vi "Acquisition.vi"(5 "Mode":enum16{"Grab", "Snap"}(ring), 6 "Image Type":T1 items=["Grayscale (U8)", "Grayscale (I16)", "Grayscale (SGL)", "Complex (CSG)", "RGB (U32)", "HSL (U32)", "RGB (U64)", "Grayscale (U16)"], 8 "Error In":errorcluster, 11 "Session In":T3) -> (0 "Error Out":errorcluster, 2 "Image Out":T2, 3 "IMAQdx Session Out":T3)   [LabVIEW 2020]
uses:
  <vilib>/userdefined/High Color/IMAQdx.ctl
  <vilib>/vision/Image Controls.llb/IMAQ Image.ctl
  <vilib>/vision/driver/IMAQdx.llb/IMAQdx Camera Control Mode.ctl
  <vilib>/vision/driver/NI_Vision_Acquisition_Software.lvlib
  <resource>/objmgr/imaqdx.rc
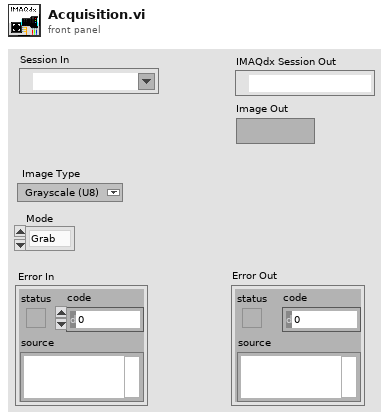
[diagram p1: front panel]
types:
  T1 = typedef "Image Type" = u32
  T2 = typedef "IMAQ Image.ctl" = refnum<image>
  T3 = typedef "IMAQdx.ctl" = refnum<k21>
  T4 = typedef "NI_Vision_Acquisition_Software.lvlib/IMAQdx Camera Control Mode.ctl" = enum32{"Controller", "Listener"}
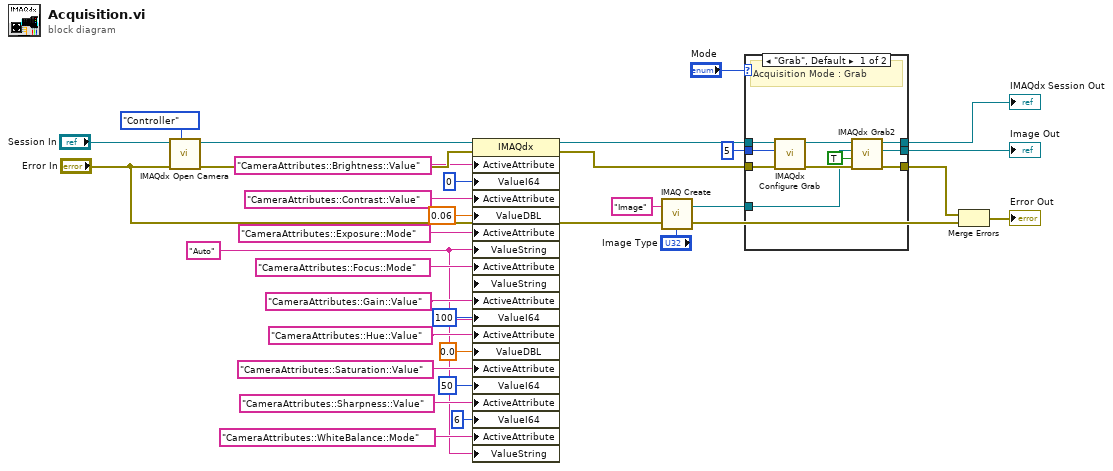
[diagram p0: block diagram]
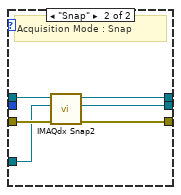
[diagram p2: hidden frame]
diagram:
  w3 = "Auto" ("ValueString")
  n1 = call <vilib>:"IMAQdx Open Camera.vi"("Camera Control Mode"=IMAQdx_Camera_Control_Mode."Controller", "error in"="Error In", "Session In"="Session In") -> ("error out"=w19:errorcluster, "Session Out"=w20:T3)  [unwired: 7 in]
  n2 = property class="IMAQdx"(reference=w20, error in=w19, "ActiveAttribute"="CameraAttributes::Brightness::Value", "ValueI64"=i64 0, "ActiveAttribute"="CameraAttributes::Contrast::Value", "ValueDBL"=0.06, "ActiveAttribute"="CameraAttributes::Exposure::Mode", "ValueString"=w3, "ActiveAttribute"="CameraAttributes::Focus::Mode", "ValueString"=w3, "ActiveAttribute"="CameraAttributes::Gain::Value", "ValueI64"=i64 100, "ActiveAttribute"="CameraAttributes::Hue::Value", "ValueDBL"=0.0, "ActiveAttribute"="CameraAttributes::Saturation::Value", "ValueI64"=i64 50, "ActiveAttribute"="CameraAttributes::Sharpness::Value", "ValueI64"=i64 6, "ActiveAttribute"="CameraAttributes::WhiteBalance::Mode", "ValueString"=w3) -> (reference out=w1:T3, error out=w2:errorcluster)
  n3 = call "IMAQ Create"("Image Name"="Image", "Image Type"="Image Type", "error in (no error)"="Error In") -> ("New Image"=w26:T2, "error out"=w30:errorcluster)  [unwired: 2 in]
  n4 = case shown="\"Grab\", Default" "Mode" {
    tunnel: u32 5 ("Number of Buffers") -> [w43 _]
    tunnel: w26 -> [w40 w44]
    tunnel: [w39 w45] -> w25
    tunnel: [w38 w47] -> w24
    tunnel: [w37 w46] -> w23
    tunnel: w1 -> [w36 w49]
    tunnel: w2 -> [w35 w48]
    frame "Grab", Default {
      # "Acquisition Mode : Grab"
      n5 = call <vilib>:"IMAQdx Configure Grab.vi"("error in"=w35, "Number of Buffers"=w43, "Session In"=w36) -> ("error out"=w41:errorcluster, "Session Out"=w42:T3)  [unwired: 7 in]
      n6 = call <vilib>:"IMAQdx Grab2.vi"("error in"=w41, "Wait for Next Buffer? (Yes)"=TRUE, "Image In"=w40, "Session In"=w42) -> ("error out"=w39:errorcluster, "Image Out"=w37:T2, "Session Out"=w38:T3)  [unwired: 4 in, 1 out]
    }
    frame "Snap" {
      # "Acquisition Mode : Snap"
      n7 = call <vilib>:"IMAQdx Snap2.vi"("error in"=w48, "Image In"=w44, "Session In"=w49) -> ("error out"=w45:errorcluster, "Image Out"=w46:T2, "Session Out"=w47:T3)  [unwired: 6 in]
    }
  }
  "IMAQdx Session Out" <- w24
  "Image Out" <- w23
  n8 = Merge Errors(w25, w30) -> (→"Error Out":errorcluster)
